vi "Logging Message Loop.vi"(8 "error in (no error)":cluster{"状态":bool, "代码":i32, "源":string} caption="错误输入（无错误）", 10 "数据队列":refnum<queue>, 11 "消息队列":T1) -> (0 "error out":cluster{"状态":bool, "代码":i32, "源":string} caption="错误输出")   [LabVIEW 2013, in "Logging.lvlib"]
doc: "消息循环子VI负责处理与记录数据相关的消息。"
uses:
  Logging.lvlib
  support/Message Queue/All Message Queues.ctl
  support/Message Queue/Message Cluster.ctl
  Logging Configuration.ctl
  Logging State.ctl
  support/Message Queue/Enqueue Message (Single).vi
  <vilib>/Utility/error.llb/Error Cluster From Error Code.vi
  <vilib>/ErrorRing/Error Ring.xnode
  support/Message Queue/Message Queue.lvlib
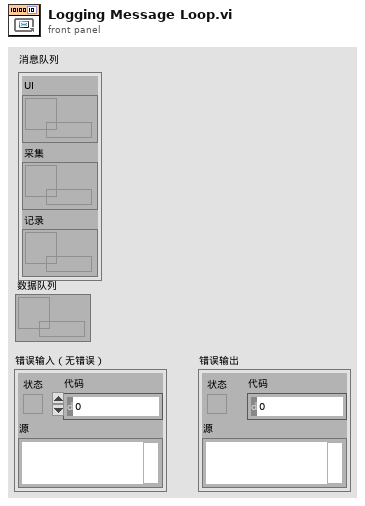
[diagram p1: front panel]
types:
  T1 = typedef "Message Queue.lvlib/All Message Queues.ctl" = cluster{"UI":refnum<queue>, "采集":refnum<queue>, "记录":refnum<queue>}
  T2 = typedef "Logging.lvlib/Logging Configuration.ctl" = cluster{"记录文件基路径":path, "TDMS文件引用":refnum<k34>}
  T3 = typedef "Logging.lvlib/Logging State.ctl" = enum16{"Idle", "Logging"}
  T4 = enum16{"open", "open or create", "create or replace", "create", "open (read-only)"}
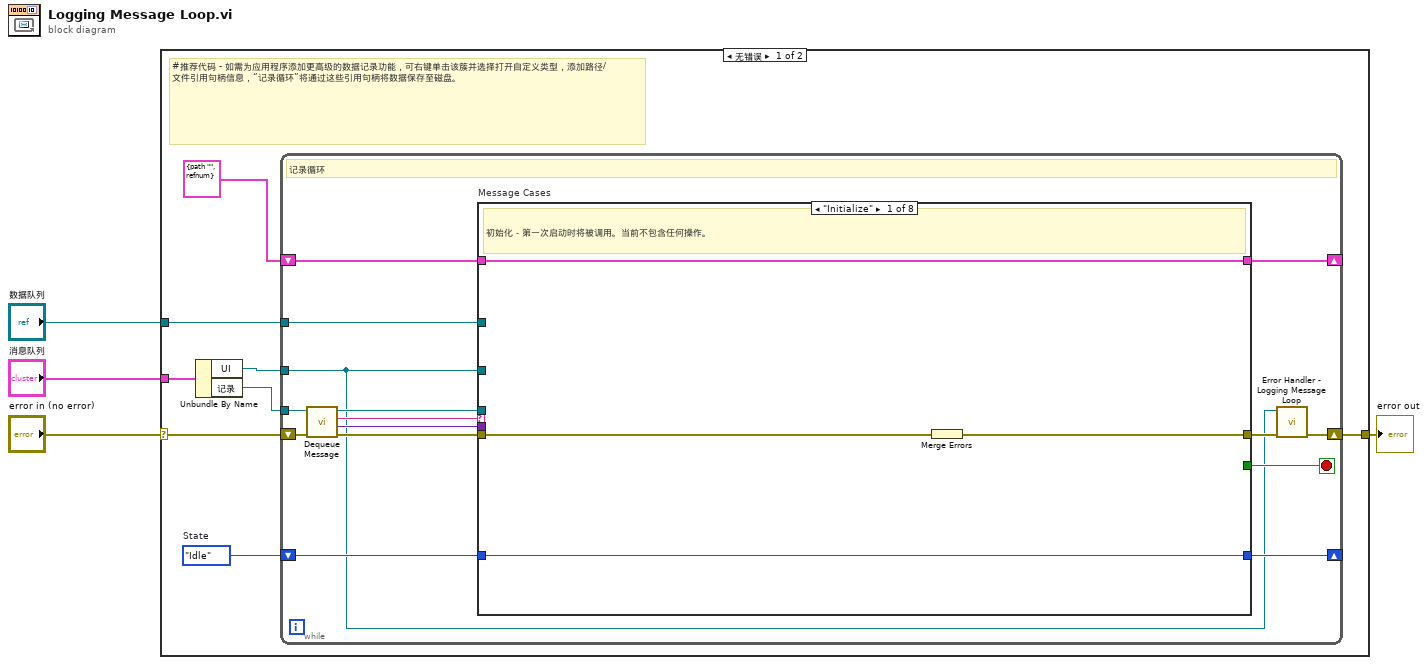
[diagram p0: block diagram]
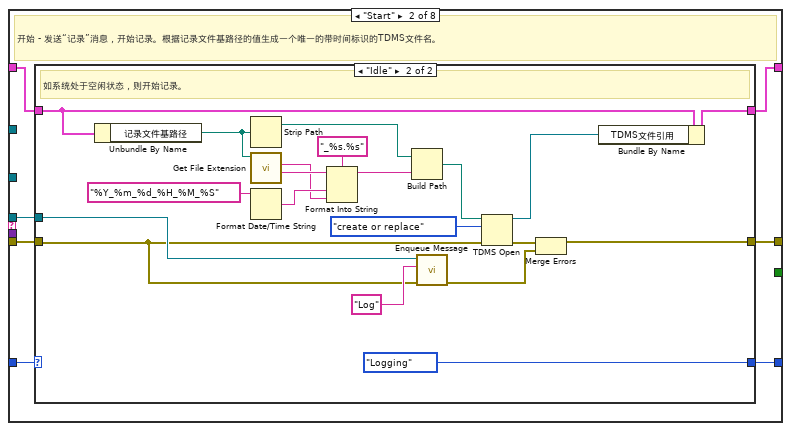
[diagram p2: hidden frame]
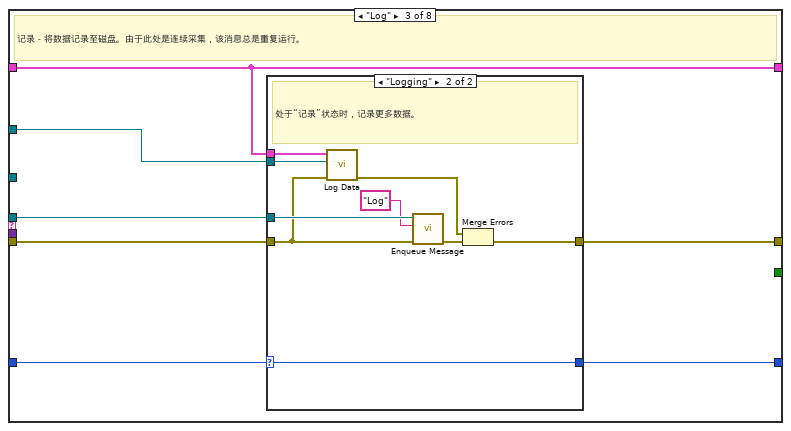
[diagram p4: hidden frame]
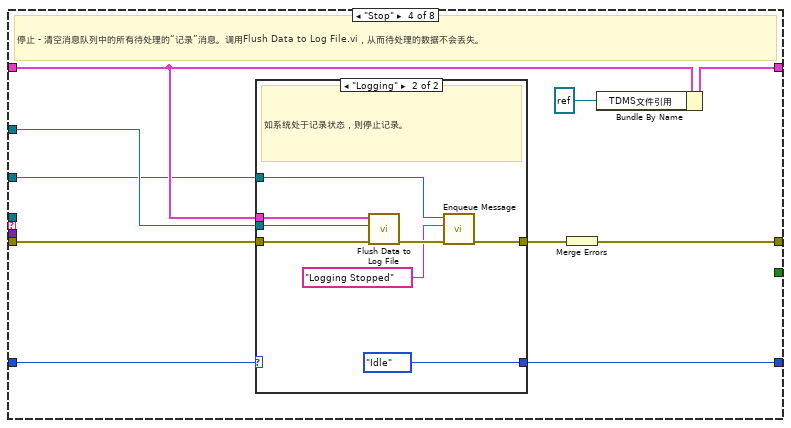
[diagram p6: hidden frame]
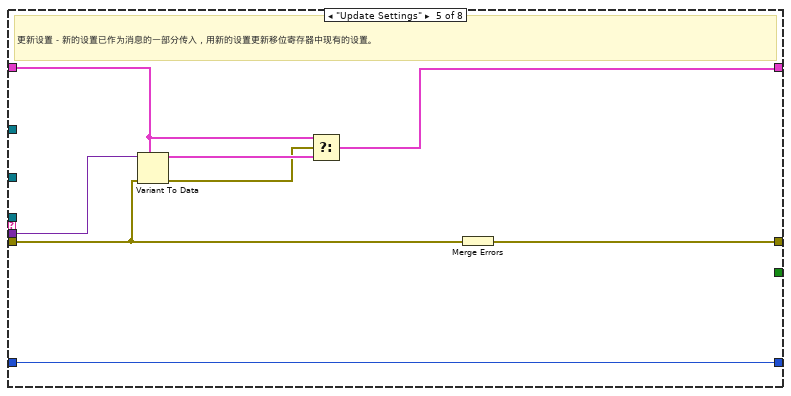
[diagram p8: hidden frame]
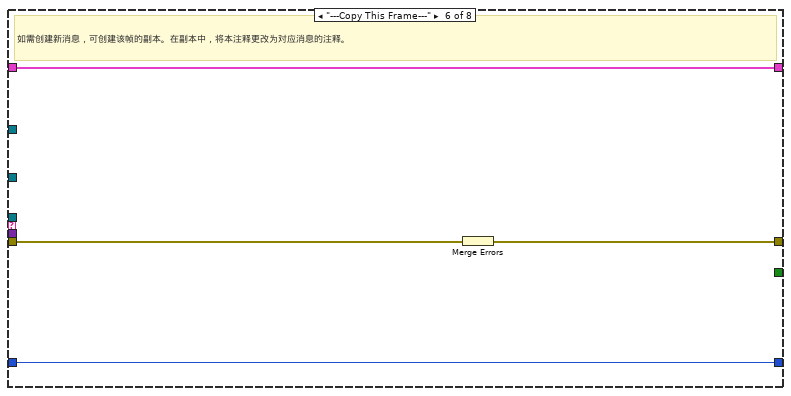
[diagram p9: hidden frame]
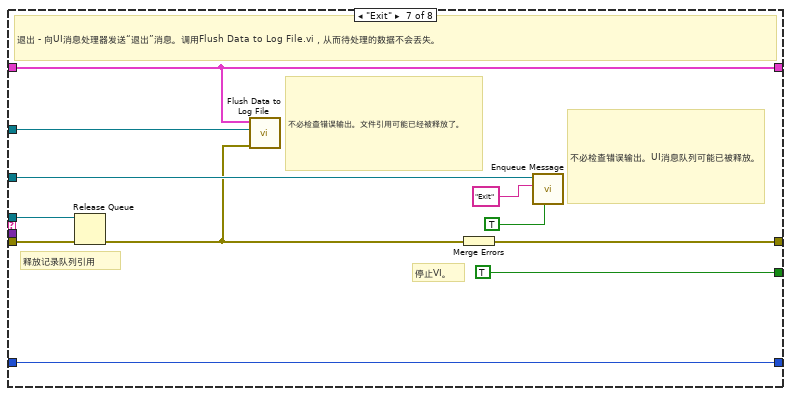
[diagram p10: hidden frame]
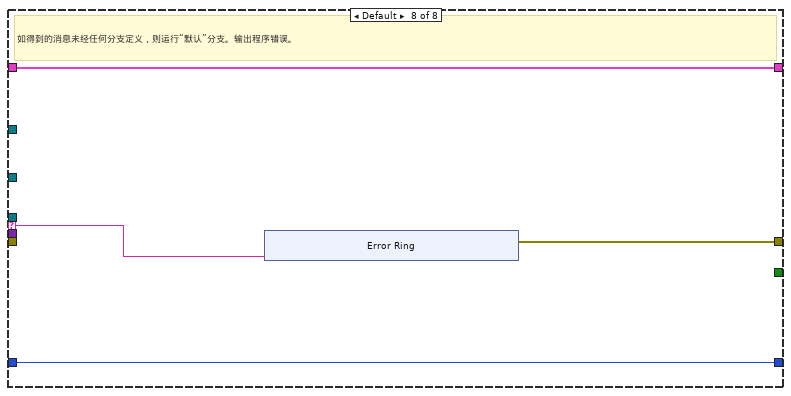
[diagram p11: hidden frame]
diagram:
  n1 = case shown="无错误" "error in (no error)" {
    selector: "error in (no error)" -> [w8 w134]
    tunnel: "消息队列" -> [w12 _]
    tunnel: [w10 w134] -> w3
    tunnel: "数据队列" -> [w7 _]
    frame No Error {
      w5 = Logging_State."Idle"  # State
      # "#推荐代码 - 如需为应用程序添加更高级的数据记录功能，可右键单击该簇并选择打开自定义类型，添加路径/文件引用句柄信息，“记录循环”将通过这些引用句柄将数据保存至磁盘。"
      n2 = Unbundle By Name(w12) -> ("UI"=w6:refnum<queue>, "记录"=w11:refnum<queue>)
      n3 = while {
        tunnel: w11 -> [w19]
        shift-right: [w26] -> _
        shift-left: T2 {"记录文件基路径"=path "", "TDMS文件引用"=refnum} ("Logging Configuration") -> [w27]
        shift-right: [w15] -> w10
        shift-left: w8 -> [w24]
        tunnel: w6 -> [w13]
        tunnel: w7 -> [w18]
        shift-right: [w16] -> _
        shift-left: w5 -> [w17]
        stop <- w25 stop-if-true
        # "记录循环"
        n4 = call "Dequeue Message.vi"("error in (no error)"=w24, "消息队列"=w19) -> ("error out"=w23:cluster{"状态":bool, "代码":i32, "源":string}, "消息数据"=w21:variant, "消息"=w22:string, "消息队列副本"=w20:refnum<queue>)  [unwired: 6 in]
        n5 = case "Message Cases" shown="\"Initialize\"" w22 {
          selector: w22 -> [_ _ _ _ _ _ _ w123]
          tunnel: w20 -> [_ w37 w67 _ _ _ w116 _]
          tunnel: w23 -> [w29 w36 w65 w83 w101 w111 w119 _]
          tunnel: [w31 w38 w68 w89 w107 w109 w121 w124] -> w14
          tunnel: w27 -> [w30 w35 w64 w84 w105 w110 w114 w126]
          tunnel: [w30 w34 w64 w87 w102 w110 w114 w126] -> w26
          tunnel: [_ _ _ _ _ _ TRUE _] -> w25
          tunnel: w21 -> [_ _ _ _ w106 _ _ _]
          tunnel: w13 -> [_ _ _ w80 _ _ w120 _]
          tunnel: w18 -> [_ _ w66 w85 _ _ w113 _]
          tunnel: w17 -> [w28 w33 w63 w82 w100 w108 w112 w125]
          tunnel: [w28 w32 w62 w81 w100 w108 w112 w125] -> w16
          frame "Initialize" {
            # "初始化－第一次启动时将被调用。当前不包含任何操作。"
            n6 = Merge Errors(w29) -> (w31:errorcluster)
          }
          frame "Start" {
            # "开始 - 发送“记录”消息，开始记录。根据记录文件基路径的值生成一个唯一的带时间标识的TDMS文件名。"
            n7 = case shown="\"Idle\"" w33 {
              selector: w33 -> [w40 _]
              tunnel: [w39 w43] -> w38
              tunnel: w37 -> [_ w44]
              tunnel: w36 -> [w39 w42]
              tunnel: w35 -> [w41 w45]
              tunnel: [w41 w47] -> w34
              tunnel: [w40 Logging_State."Logging" ("State")] -> w32
              frame "Logging" {
                # "系统已处于记录状态。忽略“开始”消息。"
              }
              frame "Idle" {
                # "如系统处于空闲状态，则开始记录。"
                n8 = Unbundle By Name(w45) -> ("记录文件基路径"=w60:path)
                n9 = Strip Path(path=w60) -> (stripped path=w57:path)  [unwired: 1 out]
                n10 = call <vilib>:"Get File Extension.vi"("file"=w60) -> ("filename without extension"=w58:string, "lowercase file extension"=w54:string)  [unwired: 7 in, 2 out]
                n11 = Format Date/Time String(time format string (%c)="%Y_%m_%d_%H_%M_%S") -> (date/time string=w55:string)  [unwired: 2 in]
                n12 = Format Into String(format string="_%s.%s", initial string=w58, w55, w54) -> (resulting string=w53:string)  [unwired: 1 in, 1 out]
                n13 = Build Path(base path=w57, name or relative path=w53) -> (appended path=w52:path)
                n14 = call-poly "Enqueue Message.vi"("error in (no error)"=w42, "消息"="Log" ("Message"), "消息队列"=w44) -> ("error out"=w50:cluster{"状态":bool, "代码":i32, "源":string})  [unwired: 7 in, 1 out]
                n15 = TDMS Open(8:w42, 10:T4."create or replace" ("operation (0:open)"), 11:w52) -> (0:w51:errorcluster, 3:w48:refnum<k34>)  [unwired: 4 in]
                n16 = Merge Errors(w51, w50) -> (w43:errorcluster)
                n17 = Bundle By Name(cluster=w45, "TDMS文件引用"=w48) -> (w47:T2)
              }
            }
          }
          frame "Log" {
            # "记录－将数据记录至磁盘。由于此处是连续采集，该消息总是重复运行。"
            n18 = case shown="\"Logging\"" w63 {
              selector: w63 -> [w70 w72]
              tunnel: [w69 w79] -> w68
              tunnel: w67 -> [_ w77]
              tunnel: w66 -> [_ w76]
              tunnel: w65 -> [w69 w71]
              tunnel: w64 -> [_ w73]
              tunnel: [w70 w72] -> w62
              frame "Idle" {
                # "如记录处于空闲状态，则忽略“记录”消息。"
              }
              frame "Logging" {
                # "处于“记录”状态时，记录更多数据。"
                n19 = call "Log Data.vi"("error in (no error)"=w71, "数据队列"=w76, "记录配置"=w73) -> ("error out"=w75:cluster{"状态":bool, "代码":i32, "源":string})  [unwired: 8 in]
                n20 = call-poly "Enqueue Message.vi"("error in (no error)"=w71, "消息"="Log" ("Message"), "消息队列"=w77) -> ("error out"=w78:cluster{"状态":bool, "代码":i32, "源":string})  [unwired: 7 in, 1 out]
                n21 = Merge Errors(w75, w78) -> (w79:errorcluster)
              }
            }
          }
          frame "Stop" {
            # "停止 - 清空消息队列中的所有待处理的“记录”消息。调用Flush Data to Log File.vi，从而待处理的数据不会丢失。"
            n22 = case shown="\"Logging\"" w82 {
              selector: w82 -> [w90 _]
              tunnel: [w91 w94] -> w88
              tunnel: w85 -> [_ w98]
              tunnel: w84 -> [_ w97]
              tunnel: w83 -> [w91 w96]
              tunnel: [w90 Logging_State."Idle" ("State")] -> w81
              tunnel: w80 -> [_ w93]
              frame "Idle" {
                # "系统已处于空闲状态。忽略“停止”消息。"
              }
              frame "Logging" {
                # "如系统处于记录状态，则停止记录。"
                n23 = call "Flush Data to Log File.vi"("error in (no error)"=w96, "数据队列"=w98, "记录配置"=w97) -> ("error out"=w99:cluster{"状态":bool, "代码":i32, "源":string})  [unwired: 8 in]
                n24 = call-poly "Enqueue Message.vi"("error in (no error)"=w99, "消息"="Logging Stopped", "消息队列"=w93) -> ("error out"=w94:cluster{"状态":bool, "代码":i32, "源":string})  [unwired: 7 in, 1 out]
              }
            }
            n25 = Merge Errors(w88) -> (w89:errorcluster)
            n26 = Bundle By Name(cluster=w84, "TDMS文件引用"=refnum<k34> refnum ("TDMS File Reference")) -> (w87:T2)
          }
          frame "Update Settings" {
            # "更新设置－新的设置已作为消息的一部分传入，用新的设置更新移位寄存器中现有的设置。"
            n27 = Variant To Data(error in=w101, type=w105, Variant=w106) -> (data=w104:T2, error out=w103:errorcluster)
            n28 = Select(t=w105, s=w103, f=w104) -> (s? t:f=w102:T2)
            n29 = Merge Errors(w101) -> (w107:errorcluster)
          }
          frame "---Copy This Frame---" {
            # "如需创建新消息，可创建该帧的副本。在副本中，将本注释更改为对应消息的注释。"
            n30 = Merge Errors(w111) -> (w109:errorcluster)
          }
          frame "Exit" {
            # "不必检查错误输出。文件引用可能已经被释放了。"
            # "释放记录队列引用"
            # "不必检查错误输出。UI消息队列可能已被释放。"
            # "停止VI。"
            # "退出 - 向UI消息处理器发送“退出”消息。调用Flush Data to Log File.vi，从而待处理的数据不会丢失。"
            n31 = Release Queue(queue=w116, error in (no error)=w119) -> (error out=w115:errorcluster)  [unwired: 1 in, 2 out]
            n32 = call "Flush Data to Log File.vi"("error in (no error)"=w115, "数据队列"=w113, "记录配置"=w114) -> ()  [unwired: 8 in, 1 out]
            n33 = Merge Errors(w115) -> (w121:errorcluster)
            n34 = call-poly "Enqueue Message.vi"("优先消息？(F)"=TRUE, "消息"="Exit" ("Message"), "消息队列"=w120) -> ()  [unwired: 7 in, 2 out]
          }
          frame Default {
            # "如得到的消息未经任何分支定义，则运行“默认”分支。输出程序错误。"
            n35 = xnode "Error Ring"("参数 0"=w123) -> ("错误输出"=w124:errorcluster)
          }
        }
        n36 = call "Error Handler - Logging Message Loop.vi"("error in (no error)"=w14, "消息队列"=w13) -> ("错误输入副本"=w15:cluster{"状态":bool, "代码":i32, "源":string})  [unwired: 8 in, 1 out]
      }
    }
    frame Error {
    }
  }
  "error out" <- w3
